vi "Square.vi"() -> (3 "Square":dynamicdata(waveform))   [LabVIEW 2018]
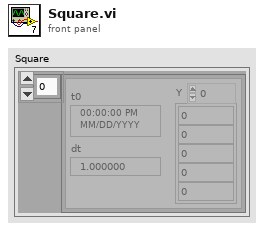
[diagram p1: front panel]
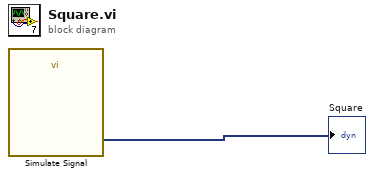
[diagram p0: block diagram]
diagram:
  n1 = call "Simulate Signal"() -> ("Square"=→"Square":dynamicdata)  [unwired: 14 in, 1 out]
